vi "KE622x -- Set Buffer Stats Params.vi"(0 "Resource In":refnum<visa-resource-name>, 1 "Check For SCPI Errors? (T)":bool=TRUE, 7 "Buffer Stats Params":T1, 11 "error in (no error)":errorcluster) -> (4 "Resource Out (dupl)":refnum<visa-resource-name>, 15 "error out":errorcluster)   [LabVIEW 2020, in "Keithley 622x.lvlib"]
doc: "Sets up the type of buffer statistics calculation the instrument will perform on readings stored in the trace buffer (Mean, Standard Deviation, Min, Max, or Peak-to-Peak), and also whether or not the statistics calculation is enabled."
uses:
  Keithley 622x.lvlib
  Typedefs/KE622x -- Buffer Stats Params.ctl
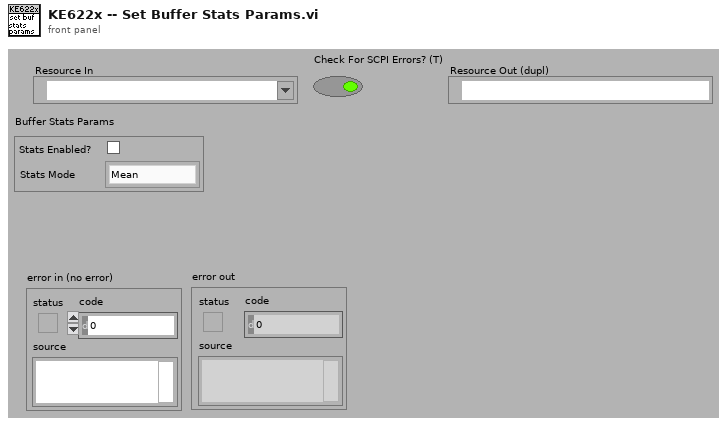
[diagram p1: front panel]
types:
  T1 = typedef "Keithley 622x.lvlib/KE622x -- Buffer Stats Params.ctl" = cluster{"Stats Enabled?":bool, "Stats Mode":enum16{"Mean", "Std Dev", "Max", "Min", "Peak-to-Peak"}}
  T2 = enum16{"Mean", "Std Dev", "Max", "Min", "Peak-to-Peak"}
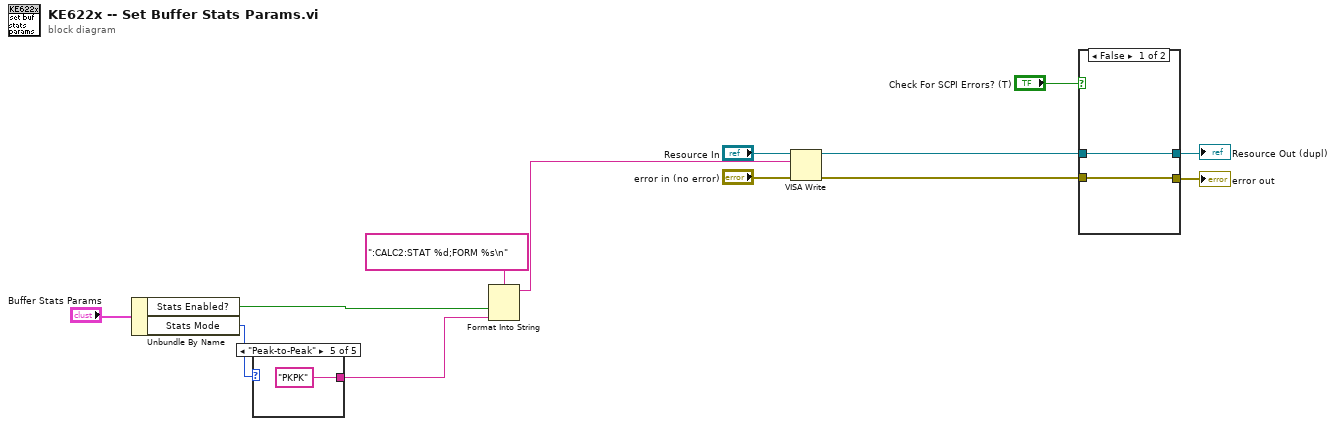
[diagram p0: block diagram]
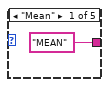
[diagram p2: hidden frame]
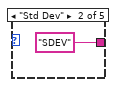
[diagram p3: hidden frame]
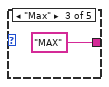
[diagram p4: hidden frame]
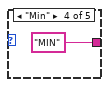
[diagram p5: hidden frame]
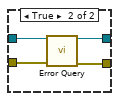
[diagram p6: hidden frame]
diagram:
  n1 = Unbundle By Name("Buffer Stats Params") -> ("Stats Enabled?"=w4:bool, "Stats Mode"=w2:T2)
  n2 = case shown="\"Peak-to-Peak\"" w2 {
    tunnel: ["MEAN" "SDEV" "MAX" "MIN" "PKPK"] -> w1
    frame "Mean" {
    }
    frame "Std Dev" {
    }
    frame "Max" {
    }
    frame "Min" {
    }
    frame "Peak-to-Peak" {
    }
  }
  n3 = Format Into String(format string=":CALC2:STAT %d;FORM %s\n", w4, w1) -> (resulting string=w3:string)  [unwired: 2 in, 1 out]
  n4 = VISA Write(VISA resource name="Resource In", write buffer=w3, error in (no error)="error in (no error)") -> (VISA resource name out=w10:refnum<visa-resource-name>, error out=w9:errorcluster)  [unwired: 1 out]
  n5 = case shown="False" "Check For SCPI Errors? (T)" {
    tunnel: w10 -> [w20 w24]
    tunnel: w9 -> [w19 w23]
    tunnel: [w19 w22] -> w7
    tunnel: [w20 w21] -> w8
    frame False {
    }
    frame True {
      n6 = call "Error Query.vi"("VISA Resource In"=w24, "error in (no error)"=w23) -> ("VISA Resource Out (dupl)"=w21:refnum<visa-resource-name>, "error out"=w22:errorcluster)  [unwired: 10 in, 2 out]
    }
  }
  "Resource Out (dupl)" <- w8
  "error out" <- w7
